vi "Create Directory.vi"(4 "Permissions":T1={"Owner"={"Read"=TRUE, "Write"=TRUE, "Execute"=TRUE}, "Group"={"Read"=TRUE, "Write"=FALSE, "Execute"=TRUE}, "Others"={"Read"=TRUE, "Write"=FALSE, "Execute"=TRUE}}, 8 "Error In":errorcluster, 10 "Remote Path":string, 11 "SFTP In":refnum<class "SFTP.lvclass">) -> (0 "Error Out":errorcluster, 3 "SFTP Out":refnum<class "SFTP.lvclass">)   [LabVIEW 2021, in "Field_RnD_Services_LIBSSH2_Toolkit.lvlib" / "SFTP.lvclass"]
doc: "Creates a directory, a.k.a. folder, on the remote SSH server."
uses:
  SFTP.lvclass
  Type Definitions/Permissions.ctl
  Type Definitions/Modes.ctl
  SFTP.lvclass/SFTP.ctl
  Field_RnD_Services_LIBSSH2_Toolkit.lvlib
  Session/Session.lvclass
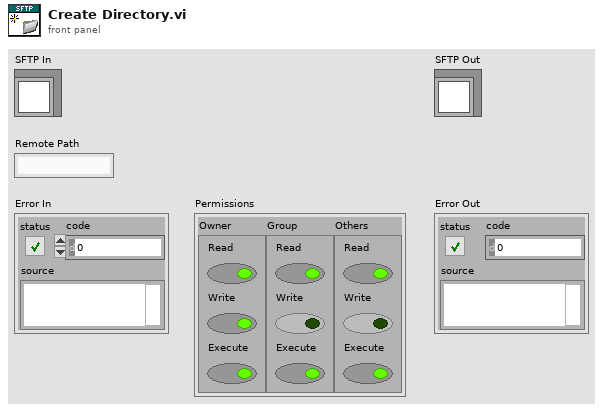
[diagram p1: front panel]
types:
  T1 = typedef "Field_RnD_Services_LIBSSH2_Toolkit.lvlib/Permissions.ctl" = cluster{"Owner":T2, "Group":T2, "Others":T2}
  T2 = typedef "Field_RnD_Services_LIBSSH2_Toolkit.lvlib/Modes.ctl" = cluster{"Read":bool, "Write":bool, "Execute":bool}
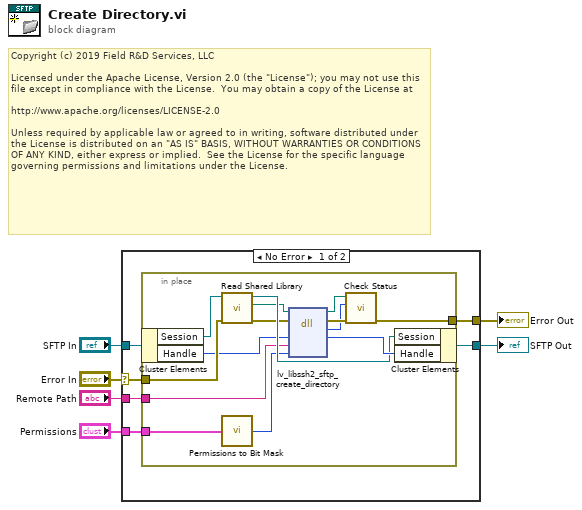
[diagram p0: block diagram]
diagram:
  # "Copyright (c) 2019 Field R&D Services, LLC\n\nLicensed under the Apache License, Version 2.0 (the \"License\"); you may not use this file except in compliance with the License.  You may obtain a copy of the License at\n\nhttp://www.apache.org/licenses/LICENSE-2.0\n\nUnless required by applicable law or agreed to in writing, software distributed under the License is distributed on an \"AS IS\" BASIS, WITHOUT WARRANTIES OR CONDITIONS OF ANY KIND, either express or implied.  See the License for the specific language governing permissions and limitations under the License."
  n1 = case shown="No Error" "Error In" {
    selector: "Error In" -> [w12 w28]
    tunnel: [w11 w28] -> w5
    tunnel: "SFTP In" -> [w10 w27]
    tunnel: [w9 w27] -> w3
    tunnel: "Remote Path" -> [w8 _]
    tunnel: "Permissions" -> [w7 _]
    frame No Error {
      n2 = in-place {
        in-place-border: w12 -> [w21]
        in-place-border: [w22] -> w11
        in-place-border: w8 -> [w15]
        in-place-border: w7 -> [w13]
        n3 = in-place-cluster #1(w10) -> ("Session"=w20:refnum<class "Session.lvclass">, "Handle"=w16:u64)
        n4 = call "Read Shared Library.vi"("Error In"=w21, "Session In"=w20) -> ("Erorr Out"=w18:errorcluster, "libssh2lv Shared Library"=w17:path, "Session Out"=w19:refnum<class "Session.lvclass">)  [unwired: 7 in]
        n5 = call "Permissions to Bit Mask.vi"("Permissions"=w13) -> ("Bit Mask"=w14:u32)
        n6 = dll-call lib="libssh2lv.*" fn="lv_libssh2_sftp_create_directory"(path in=w17, error in=w18, "handle"=w16, "directory_path"=w15, "mode"=w14) -> (path out=w24:path, error out=w25:errorcluster, "status"=w23:i32, "handle"=w26:u64)  [unwired: 3 in]
        n7 = call "Check Status.vi"("Error In"=w25, "Status"=w23, "libssh2lv Shared Library In"=w24) -> ("Error Out"=w22:errorcluster)  [unwired: 7 in, 1 out]
        n8 = in-place-cluster #1("Session"=w19, "Handle"=w26) -> (w9:refnum<class "SFTP.lvclass">)
      }
    }
    frame Error {
    }
  }
  "Error Out" <- w5
  "SFTP Out" <- w3
